vi "Create Axis Labels.vi"(4 "Inverted":bool, 5 "Range":cluster{"Max":sgl, "Min":sgl}, 6 "Font Color":u32(colorbox), 7 "Which Axis?":T1(ring)=enum."Z Opposite", 8 "error in (no error)":errorcluster, 9 "Font Size":u16, 10 "Alpha":sgl, 11 "Tick Cluster Array":T2) -> (0 "error out":errorcluster, 1 "Max Width":sgl, 3 "New Label Object":refnum<vi>)   [LabVIEW 2017, in "3D Plot.lvclass"]
uses:
  <vilib>/Math Plots/3D Math Plots/3D Plot/3D Plot/3D Plot.lvclass
  <vilib>/Math Plots/3D Math Plots/3D Plot/3D Plot/Typedef/Tick Array.ctl
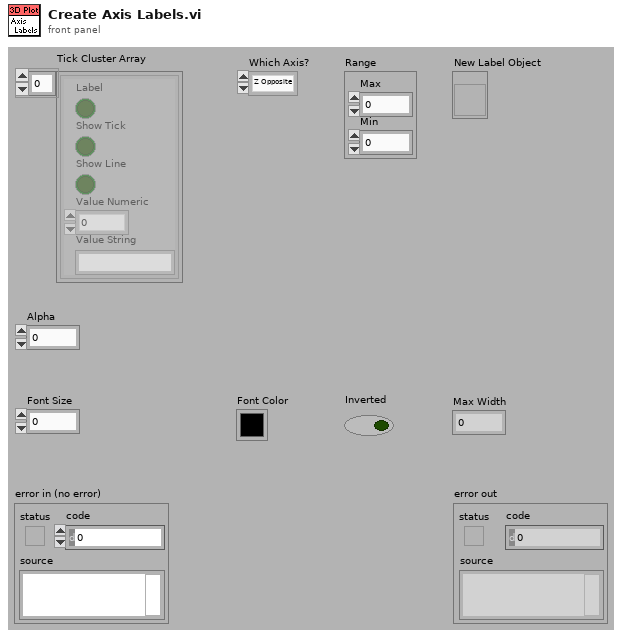
[diagram p1: front panel]
types:
  T1 = enum16{"X", "Y", "Z", "X Opposite", "Y Opposite", "Z Opposite"}
  T2 = typedef "3D Plot.lvclass/Tick Array.ctl" = cluster{"Label":bool, "Show Tick":bool, "Show Line":bool, "Value Numeric":sgl, "Value String":string}[]
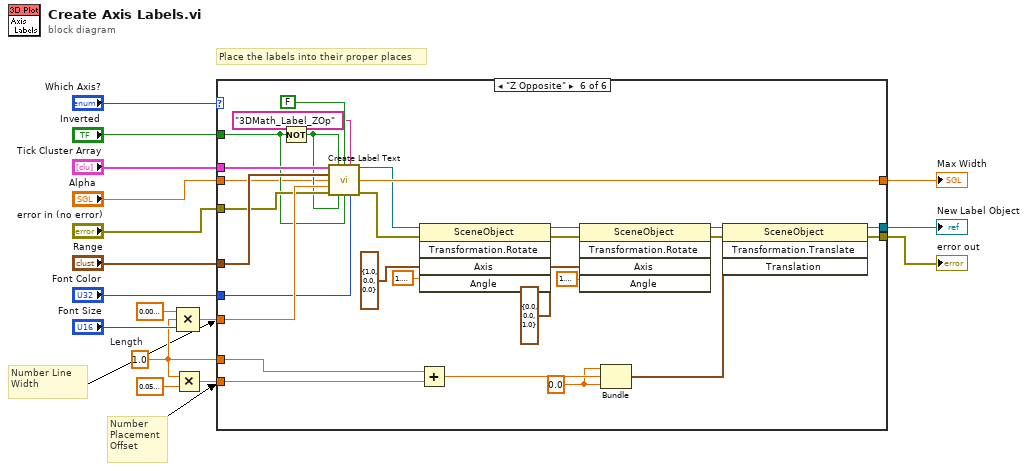
[diagram p0: block diagram]
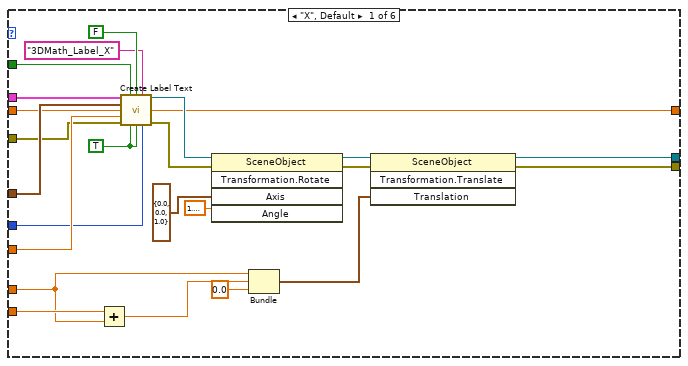
[diagram p2: hidden frame]
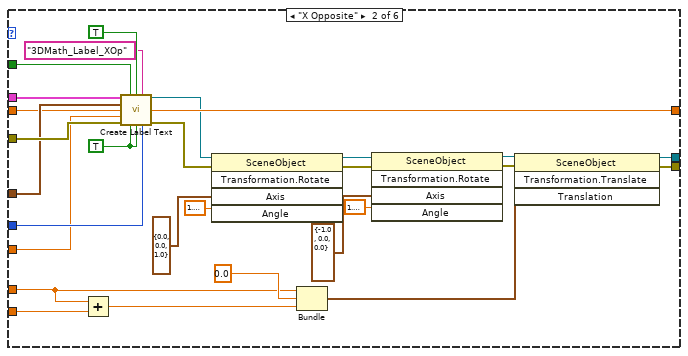
[diagram p3: hidden frame]
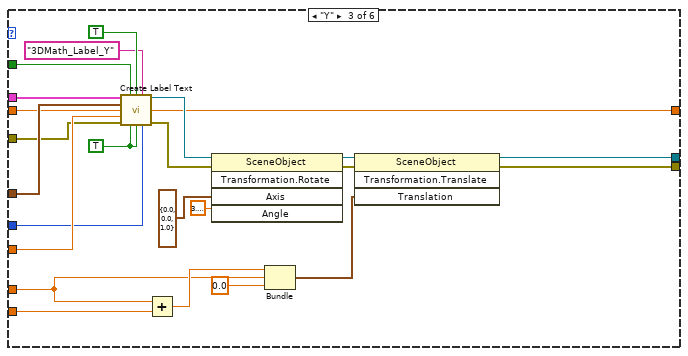
[diagram p4: hidden frame]
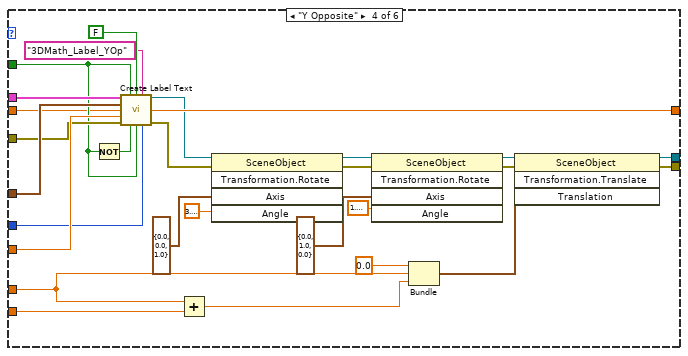
[diagram p5: hidden frame]
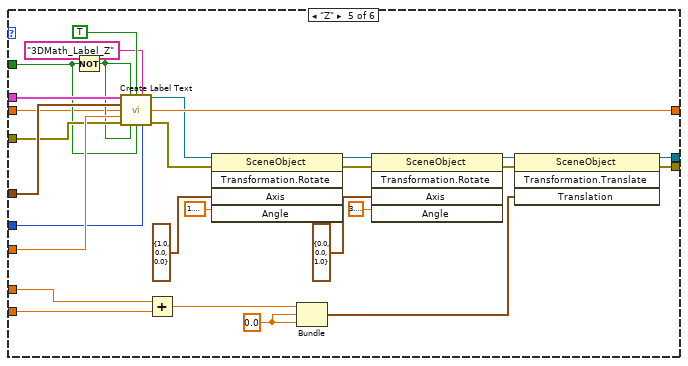
[diagram p6: hidden frame]
diagram:
  w2 = sgl 1.0  # Length
  # "Place the labels into their proper places"
  # "Number \nPlacement\nOffset"
  # "Number Line\nWidth"
  n1 = Multiply(x=w2, y=sgl 0.06) -> (x*y=w6:sgl)
  n2 = Compound Arithmetic op=MULTIPLY(sgl 0.01, w2, "Font Size") -> (w7:sgl)
  n3 = case shown="\"Z Opposite\"" "Which Axis?" {
    tunnel: w2 -> [w28 w47 w80 w103 w132 w160]
    tunnel: [w37 w66 w86 w118 w144 w173] -> w13
    tunnel: w6 -> [w34 w58 w85 w110 w138 w169]
    tunnel: w7 -> [w27 w48 w79 w102 w131 w159]
    tunnel: "Font Color" -> [w25 w53 w76 w100 w128 w156]
    tunnel: [w21 w52 w71 w98 w126 w154] -> w15
    tunnel: "Tick Cluster Array" -> [w30 w45 w82 w105 w134 w162]
    tunnel: "Range" -> [w29 w46 w81 w104 w133 w161]
    tunnel: "Inverted" -> [w24 w44 w74 w95 w129 w157]
    tunnel: [w31 w55 w83 w107 w135 w163] -> w10
    tunnel: "error in (no error)" -> [w26 w49 w78 w101 w130 w158]
    tunnel: "Alpha" -> [w17 w41 w69 w93 w121 w149]
    frame "X", Default {
      w19 = TRUE ("Draw First Label?")
      n4 = Add(x=w34, y=w28) -> (x+y=w35:sgl)
      n5 = call <vilib>:"Create Label Text.vi"("Tick Cluster Array"=w30, "Reverse?"=w24, "Right justified"=FALSE, "Label Object Name"="3DMath_Label_X", "Range"=w29, "Alpha"=w17, "Width"=w27, "error in (no error)"=w26, "Draw Last Label?"=w19, "Draw First Label?"=w19, "Color Box"=w25) -> ("New Label Object"=w22:refnum<vi>, "Max Width"=w21:sgl, "error out"=w20:errorcluster)  [unwired: 2 out]
      n6 = invoke class="SceneObject" method="Transformation.Rotate"(reference=w22, error in=w20, "Axis"=cluster{"X":sgl, "Y":sgl, "Z":sgl} {"X"=0.0, "Y"=0.0, "Z"=1.0}, "Angle"=sgl 1.5707964) -> (reference out=w33:refnum<vi>, error out=w32:errorcluster)  [unwired: 1 in, 3 out]
      n7 = Bundle("Length"=w28, w35, "Z"=sgl 0.0) -> (w38:cluster{"Length":sgl, sgl, "Z":sgl})  [unwired: 1 out]
      n8 = invoke class="SceneObject" method="Transformation.Translate"(reference=w33, error in=w32, "Translation"=w38) -> (reference out=w37:refnum<vi>, error out=w31:errorcluster)  [unwired: 1 in, 2 out]
    }
    frame "X Opposite" {
      w54 = TRUE ("Draw First Label?")
      n9 = Add(x=w47, y=w58) -> (x+y=w60:sgl)
      n10 = call <vilib>:"Create Label Text.vi"("Tick Cluster Array"=w45, "Reverse?"=w44, "Right justified"=TRUE, "Label Object Name"="3DMath_Label_XOp", "Range"=w46, "Alpha"=w41, "Width"=w48, "error in (no error)"=w49, "Draw Last Label?"=w54, "Draw First Label?"=w54, "Color Box"=w53) -> ("New Label Object"=w51:refnum<vi>, "Max Width"=w52:sgl, "error out"=w50:errorcluster)  [unwired: 2 out]
      n11 = invoke class="SceneObject" method="Transformation.Rotate"(reference=w51, error in=w50, "Axis"=cluster{"X":sgl, "Y":sgl, "Z":sgl} {"X"=0.0, "Y"=0.0, "Z"=1.0}, "Angle"=sgl 1.5707964) -> (reference out=w64:refnum<vi>, error out=w57:errorcluster)  [unwired: 1 in, 3 out]
      n12 = Bundle("Length"=w47, "Z"=sgl 0.0, w60) -> (w67:cluster{"Length":sgl, "Z":sgl, sgl})  [unwired: 1 out]
      n13 = invoke class="SceneObject" method="Transformation.Rotate"(reference=w64, error in=w57, "Axis"=cluster{"X":sgl, "Y":sgl, "Z":sgl} {"X"=-1.0, "Y"=0.0, "Z"=0.0}, "Angle"=sgl 1.5707964) -> (reference out=w63:refnum<vi>, error out=w56:errorcluster)  [unwired: 1 in, 3 out]
      n14 = invoke class="SceneObject" method="Transformation.Translate"(reference=w63, error in=w56, "Translation"=w67) -> (reference out=w66:refnum<vi>, error out=w55:errorcluster)  [unwired: 1 in, 2 out]
    }
    frame "Y" {
      w75 = TRUE ("Draw First Label?")
      n15 = call <vilib>:"Create Label Text.vi"("Tick Cluster Array"=w82, "Reverse?"=w74, "Right justified"=TRUE, "Label Object Name"="3DMath_Label_Y", "Range"=w81, "Alpha"=w69, "Width"=w79, "error in (no error)"=w78, "Draw Last Label?"=w75, "Draw First Label?"=w75, "Color Box"=w76) -> ("New Label Object"=w72:refnum<vi>, "Max Width"=w71:sgl, "error out"=w77:errorcluster)  [unwired: 2 out]
      n16 = Add(x=w80, y=w85) -> (x+y=w90:sgl)
      n17 = invoke class="SceneObject" method="Transformation.Rotate"(reference=w72, error in=w77, "Axis"=cluster{"X":sgl, "Y":sgl, "Z":sgl} {"X"=0.0, "Y"=0.0, "Z"=1.0}, "Angle"=sgl 3.1415927) -> (reference out=w89:refnum<vi>, error out=w84:errorcluster)  [unwired: 1 in, 3 out]
      n18 = Bundle(w90, "Length"=w80, "Z"=sgl 0.0) -> (w87:cluster{sgl, "Length":sgl, "Z":sgl})  [unwired: 1 out]
      n19 = invoke class="SceneObject" method="Transformation.Translate"(reference=w89, error in=w84, "Translation"=w87) -> (reference out=w86:refnum<vi>, error out=w83:errorcluster)  [unwired: 1 in, 2 out]
    }
    frame "Y Opposite" {
      n20 = Not(x=w95) -> (.not. x?=w106:bool)
      n21 = call <vilib>:"Create Label Text.vi"("Tick Cluster Array"=w105, "Reverse?"=w95, "Right justified"=FALSE, "Label Object Name"="3DMath_Label_YOp", "Range"=w104, "Alpha"=w93, "Width"=w102, "error in (no error)"=w101, "Draw Last Label?"=w106, "Draw First Label?"=w95, "Color Box"=w100) -> ("New Label Object"=w97:refnum<vi>, "Max Width"=w98:sgl, "error out"=w99:errorcluster)  [unwired: 2 out]
      n22 = Add(x=w103, y=w110) -> (x+y=w111:sgl)
      n23 = invoke class="SceneObject" method="Transformation.Rotate"(reference=w97, error in=w99, "Axis"=cluster{"X":sgl, "Y":sgl, "Z":sgl} {"X"=0.0, "Y"=0.0, "Z"=1.0}, "Angle"=sgl 3.1415927) -> (reference out=w117:refnum<vi>, error out=w109:errorcluster)  [unwired: 1 in, 3 out]
      n24 = invoke class="SceneObject" method="Transformation.Rotate"(reference=w117, error in=w109, "Axis"=cluster{"X":sgl, "Y":sgl, "Z":sgl} {"X"=0.0, "Y"=1.0, "Z"=0.0}, "Angle"=sgl 1.5707964) -> (reference out=w116:refnum<vi>, error out=w108:errorcluster)  [unwired: 1 in, 3 out]
      n25 = Bundle("Z"=sgl 0.0, "Length"=w103, w111) -> (w119:cluster{"Z":sgl, "Length":sgl, sgl})  [unwired: 1 out]
      n26 = invoke class="SceneObject" method="Transformation.Translate"(reference=w116, error in=w108, "Translation"=w119) -> (reference out=w118:refnum<vi>, error out=w107:errorcluster)  [unwired: 1 in, 2 out]
    }
    frame "Z" {
      w139 = sgl 0.0 ("Z")
      n27 = Not(x=w129) -> (.not. x?=w123:bool)
      n28 = call <vilib>:"Create Label Text.vi"("Tick Cluster Array"=w134, "Reverse?"=w123, "Right justified"=TRUE, "Label Object Name"="3DMath_Label_Z", "Range"=w133, "Alpha"=w121, "Width"=w131, "error in (no error)"=w130, "Draw Last Label?"=w123, "Draw First Label?"=w129, "Color Box"=w128) -> ("New Label Object"=w125:refnum<vi>, "Max Width"=w126:sgl, "error out"=w127:errorcluster)  [unwired: 2 out]
      n29 = Add(x=w132, y=w138) -> (x+y=w147:sgl)
      n30 = invoke class="SceneObject" method="Transformation.Rotate"(reference=w125, error in=w127, "Axis"=cluster{"X":sgl, "Y":sgl, "Z":sgl} {"X"=1.0, "Y"=0.0, "Z"=0.0}, "Angle"=sgl 1.5707964) -> (reference out=w143:refnum<vi>, error out=w137:errorcluster)  [unwired: 1 in, 3 out]
      n31 = Bundle(w147, "Z"=w139, "Z"=w139) -> (w145:cluster{sgl, "Z":sgl, "Z":sgl})  [unwired: 1 out]
      n32 = invoke class="SceneObject" method="Transformation.Rotate"(reference=w143, error in=w137, "Axis"=cluster{"X":sgl, "Y":sgl, "Z":sgl} {"X"=0.0, "Y"=0.0, "Z"=1.0}, "Angle"=sgl 3.1415927) -> (reference out=w142:refnum<vi>, error out=w136:errorcluster)  [unwired: 1 in, 3 out]
      n33 = invoke class="SceneObject" method="Transformation.Translate"(reference=w142, error in=w136, "Translation"=w145) -> (reference out=w144:refnum<vi>, error out=w135:errorcluster)  [unwired: 1 in, 2 out]
    }
    frame "Z Opposite" {
      w167 = sgl 0.0 ("Z")
      n34 = Not(x=w157) -> (.not. x?=w151:bool)
      n35 = call <vilib>:"Create Label Text.vi"("Tick Cluster Array"=w162, "Reverse?"=w151, "Right justified"=FALSE, "Label Object Name"="3DMath_Label_ZOp", "Range"=w161, "Alpha"=w149, "Width"=w159, "error in (no error)"=w158, "Draw Last Label?"=w151, "Draw First Label?"=w157, "Color Box"=w156) -> ("New Label Object"=w153:refnum<vi>, "Max Width"=w154:sgl, "error out"=w155:errorcluster)  [unwired: 2 out]
      n36 = Add(x=w160, y=w169) -> (x+y=w168:sgl)
      n37 = invoke class="SceneObject" method="Transformation.Rotate"(reference=w153, error in=w155, "Axis"=cluster{"X":sgl, "Y":sgl, "Z":sgl} {"X"=1.0, "Y"=0.0, "Z"=0.0}, "Angle"=sgl 1.5707964) -> (reference out=w172:refnum<vi>, error out=w165:errorcluster)  [unwired: 1 in, 3 out]
      n38 = invoke class="SceneObject" method="Transformation.Rotate"(reference=w172, error in=w165, "Axis"=cluster{"X":sgl, "Y":sgl, "Z":sgl} {"X"=0.0, "Y"=0.0, "Z"=1.0}, "Angle"=sgl 1.5707964) -> (reference out=w171:refnum<vi>, error out=w164:errorcluster)  [unwired: 1 in, 3 out]
      n39 = Bundle("Z"=w167, w168, "Z"=w167) -> (w174:cluster{"Z":sgl, sgl, "Z":sgl})  [unwired: 1 out]
      n40 = invoke class="SceneObject" method="Transformation.Translate"(reference=w171, error in=w164, "Translation"=w174) -> (reference out=w173:refnum<vi>, error out=w163:errorcluster)  [unwired: 1 in, 2 out]
    }
  }
  "error out" <- w10
  "New Label Object" <- w13
  "Max Width" <- w15
